vi "initialize.vi"(0 "HGF_Notifier":refnum<class "HGF_Notifier.lvclass">, 3 "initializationData":variant, 5 "error in (no error)":errorcluster, 7 "binaryString":string, 8 "I8 Array":i8[](array[numeric]), 9 "prependSize? (T)":bool, 11 "byteOrder (0:big-endian, network order)":T1(ring)) -> (14 "dup HGF_Notifier":refnum<class "HGF_Notifier.lvclass">, 17 "found?":bool, 19 "error out":errorcluster)   [LabVIEW 2014, in "HGF_BaseClasses.lvlib" / "HGF_Notifier.lvclass"]
doc: "This is a dynamic dispatch VI to be implemented by child classes to initialize their attributes.\n\n<B>Recommendation:</B> Use Variant for initialization data."
uses:
  HGF_Notifier.lvclass
  HGF_TriggeredEvent/HGF_TriggeredEvent.lvclass
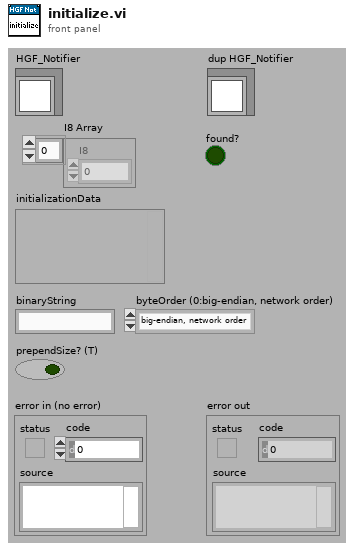
[diagram p1: front panel]
types:
  T1 = enum16{"big-endian, network order", "native, host order", "little-endian"}
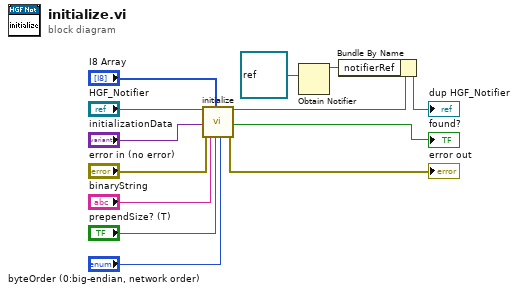
[diagram p0: block diagram]
diagram:
  n1 = call-parent "initialize.vi"("HGF_Timing"="HGF_Notifier", "initializationData"="initializationData", "error in (no error)"="error in (no error)", "binaryString"="binaryString", "I8 Array"="I8 Array", "prependSize? (T)"="prependSize? (T)", "byteOrder (0:big-endian, network order)"="byteOrder (0:big-endian, network order)") -> ("dup HGF_Timing"=w6:refnum<class "HGF_Notifier.lvclass">, "found?"=→"found?":bool, "error out"=→"error out":errorcluster)  [unwired: 1 in, 9 out]
  n2 = Obtain Notifier(notification data type=refnum<class> refnum ("LabVIEW Object")) -> (notifier out=w4:refnum<notifier>)  [unwired: 2 in, 3 out]
  n3 = Bundle By Name(cluster=w6, "notifierRef"=w4) -> (→"dup HGF_Notifier":refnum<class "HGF_Notifier.lvclass">)
